vi "svx_Waterfall Execute.vi"(0 "Data In":T2={"z0"=0.0, "dz"=1.0, "Plots"=[]}, 1 "Display State In":T6={"X Scale Width %"=50.0, "Y Scale Height %"=50.0, "X-Axis Range"={"Minimum"=0.0, "Maximum"=10.0}, "Y-Axis Range"={"Minimum"=0.0, "Maximum"=10.0}, "Z-Axis Range"={"Minimum"=0.0, "Maximum"=10.0}, "Plot Color"=61212, "Frame Color"=16252785, "Background Color"=16777222, "Initial AutoScale Y"=TRUE, "AutoScale X"=2, "AutoScale Y"=2, "AutoScale Z"=2, "Plot Transparency"=FALSE, "X-Axis Name"="Frequency", "Y-Axis Name"="Amplitude", "Z-Axis Name"="", "X-Axis Scaling Factor"={"Offset"=0.0, "Multiplier"=1.0}, "Y-Axis Scaling Factor"={"Offset"=0.0, "Multiplier"=1.0}, "Z-Axis Scaling Factor"={"Offset"=0.0, "Multiplier"=1.0}, "X-Scale Visible"=TRUE, "Y-Scale Visible"=TRUE, "Z-Scale Visible"=TRUE, "X-Scale Label Visible"=TRUE, "Y-Scale Label Visible"=TRUE, "Z-Scale Label Visible"=TRUE, "X-Axis Range Scaled"={"Minimum"=0.0, "Maximum"=10.0}, "Y-Axis Range Scaled"={"Minimum"=0.0, "Maximum"=10.0}, "Z-Axis Range Scaled"={"Minimum"=0.0, "Maximum"=10.0}, "Rev Z Order"=FALSE, "X-Scale Format Str"="%#.4g", "Y-Scale Format Str"="%#.4g", "Z-Scale Format Str"="%#.4g", "Decor color"=12369084, "Scale Range Change"=refnum, "out of state queue"=refnum, "property nodes"=refnum, "Lines"=[], "Line Properties"={"Line Color"=61212, "Line Width"=61212, "Line Style"=enum."Dash", "DisplayLines"=FALSE}} {"Line Properties"."Line Width" min=1}, 2 "Container State":T7, 4 "Dec/Cropped and Lines":T1={"Dec/Cropped in"={"z0"=0.0, "dz"=1.0, "Plots"=[]}, "Lines"=[]}, 6 "Execution Tasks":T5[](array[typedef]), 7 "XY Graph Ref":refnum<vi>, 8 "Coords":T4, 9 "XY Scale Graph ref":refnum<vi>, 11 "Z Scale Graph ref":refnum<vi>, 12 "This VI":refnum<vi>, 13 "Background ref":refnum<vi>) -> (14 "Data Out":T2={"z0"=0.0, "dz"=1.0, "Plots"=[]}, 15 "Display State Out":T6={"X Scale Width %"=50.0, "Y Scale Height %"=50.0, "X-Axis Range"={"Minimum"=0.0, "Maximum"=10.0}, "Y-Axis Range"={"Minimum"=0.0, "Maximum"=10.0}, "Z-Axis Range"={"Minimum"=0.0, "Maximum"=10.0}, "Plot Color"=61212, "Frame Color"=16252785, "Background Color"=16777222, "Initial AutoScale Y"=TRUE, "AutoScale X"=2, "AutoScale Y"=2, "AutoScale Z"=2, "Plot Transparency"=FALSE, "X-Axis Name"="Frequency", "Y-Axis Name"="Amplitude", "Z-Axis Name"="", "X-Axis Scaling Factor"={"Offset"=0.0, "Multiplier"=1.0}, "Y-Axis Scaling Factor"={"Offset"=0.0, "Multiplier"=1.0}, "Z-Axis Scaling Factor"={"Offset"=0.0, "Multiplier"=1.0}, "X-Scale Visible"=TRUE, "Y-Scale Visible"=TRUE, "Z-Scale Visible"=TRUE, "X-Scale Label Visible"=TRUE, "Y-Scale Label Visible"=TRUE, "Z-Scale Label Visible"=TRUE, "X-Axis Range Scaled"={"Minimum"=0.0, "Maximum"=10.0}, "Y-Axis Range Scaled"={"Minimum"=0.0, "Maximum"=10.0}, "Z-Axis Range Scaled"={"Minimum"=0.0, "Maximum"=10.0}, "Rev Z Order"=FALSE, "X-Scale Format Str"="%#.4g", "Y-Scale Format Str"="%#.4g", "Z-Scale Format Str"="%#.4g", "Decor color"=12369084, "Scale Range Change"=refnum, "out of state queue"=refnum, "property nodes"=refnum, "Lines"=[], "Line Properties"={"Line Color"=61212, "Line Width"=61212, "Line Style"=enum."Dash", "DisplayLines"=FALSE}} {"Line Properties"."Line Width" min=1}, 18 "Dec/Cropped out":T1={"Dec/Cropped in"={"z0"=0.0, "dz"=1.0, "Plots"=[]}, "Lines"=[]})   [LabVIEW 2017, in "SVX Waterfall Graph.xctl"]
uses:
  <vilib>/addons/_XControls/Waterfall Graph/SVX Waterfall Graph.xctl
  <vilib>/addons/_XControls/Waterfall Graph/subVIs/svx_Waterfall State.ctl
  <vilib>/addons/_NISVFA/_Shared subVIs/Controls/svc_Cluster of Array of Cluster of XYZ.ctl
  <vilib>/_xctls/Container State.ctl
  <vilib>/addons/_XControls/Waterfall Graph/subVIs/svx_Waterfall Data.ctl
  <vilib>/addons/_XControls/Waterfall Graph/subVIs/svx_Waterfall Execution Tasks.ctl
  <vilib>/Utility/miscctls.llb/LVPoint32TypeDef.ctl
  <vilib>/addons/_XControls/Waterfall Graph/subVIs/svx_CroppedData.ctl
  <vilib>/_xctls/XControlSupport.lvlib
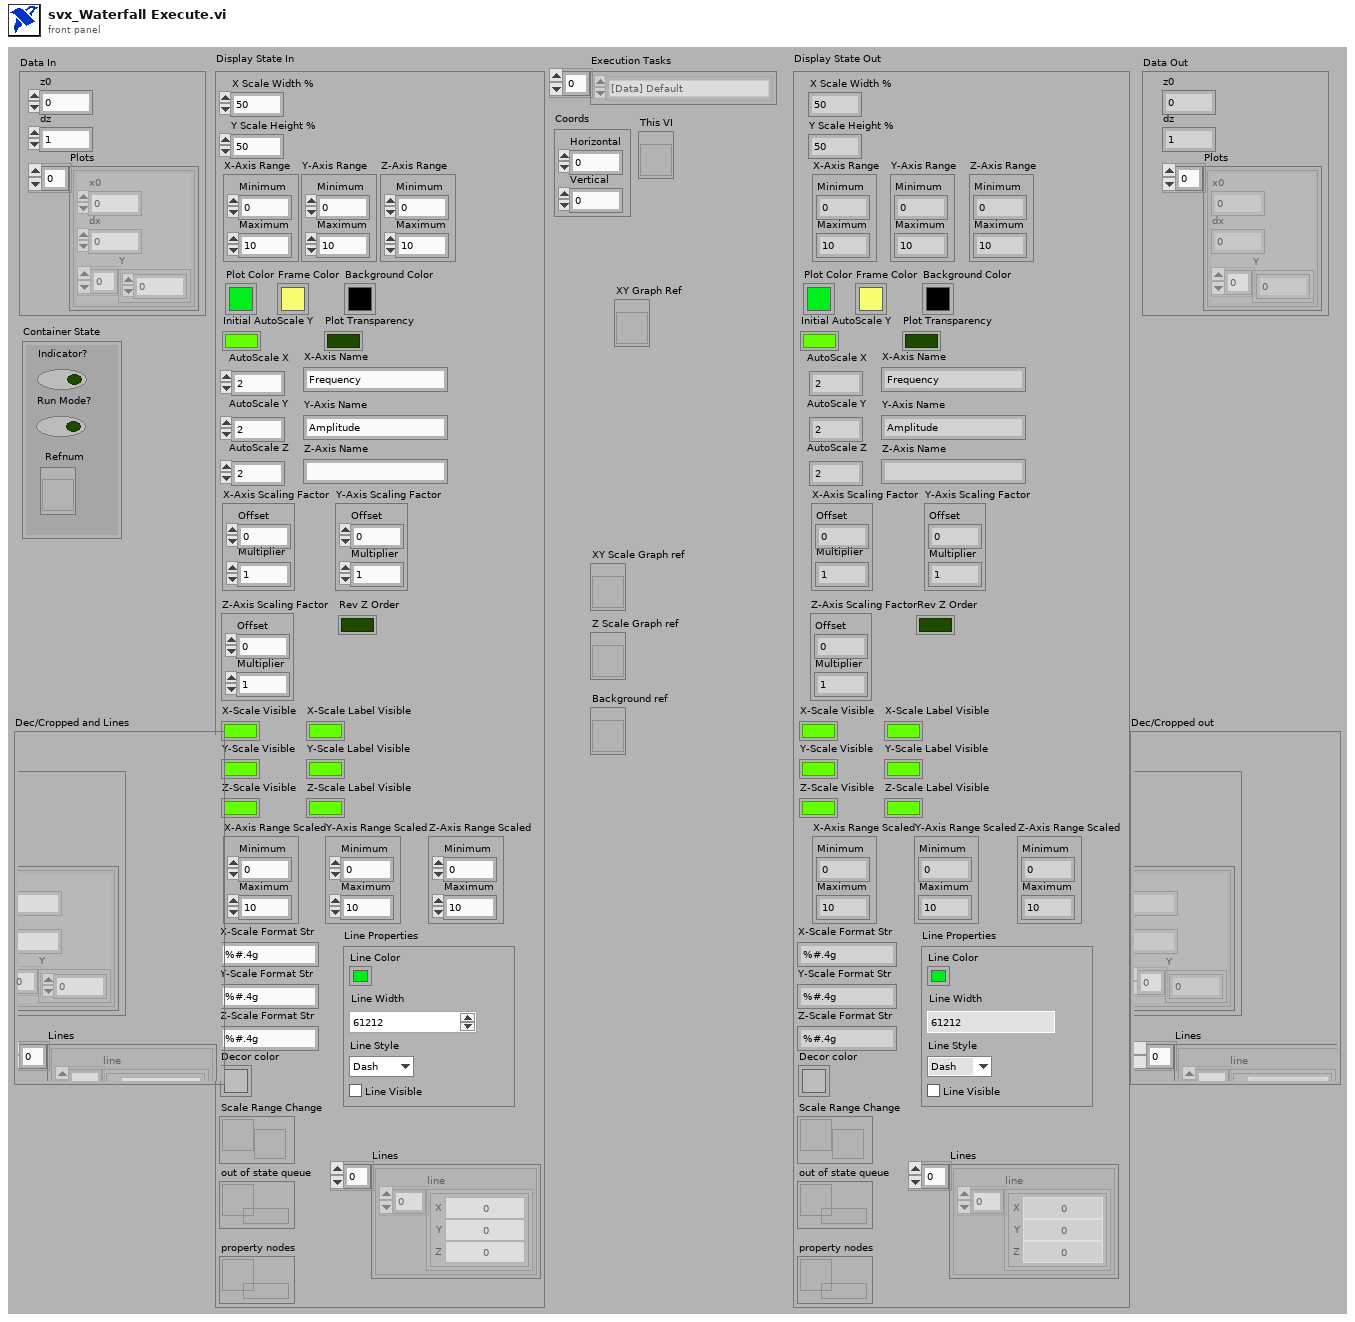
[diagram p1: front panel]
types:
  T1 = typedef "SVX Waterfall Graph.xctl/svx_CroppedData.ctl" = cluster{"Dec/Cropped in":T2, "Lines":T3[]}
  T2 = typedef "SVX Waterfall Graph.xctl/svx_Waterfall Data.ctl" = cluster{"z0":dbl, "dz":dbl, "Plots":cluster{"x0":dbl, "dx":dbl, "Y":dbl[]}[]}
  T3 = typedef "svc_Cluster of Array of Cluster of XYZ.ctl" = cluster{"line":cluster{"X":dbl, "Y":dbl, "Z":dbl}[]}
  T4 = typedef "LVPoint32TypeDef.ctl" = cluster{"Horizontal":i32, "Vertical":i32}
  T5 = typedef "SVX Waterfall Graph.xctl/svx_Waterfall Execution Tasks.ctl" = enum16{"[Data] Default", "[Data] Update Graph", "[Pane] Calculate Size from Coord Change", "[Pane] Calculate Size from Display State", "[Plot] Redraw Frame", "[Plot] Update Plot Color", "[Scale] Autoscale or Crop X, Y, Z", "[Scale] Resize Scales", "[Scale] Align Scale Labels", "[Plot] Initialize Plot", "[Scale] X Scale", "[Scale] Y Scale", "[Scale] Z Scale", "[Scale] Multiplier/Offset", "[Scale] Name", "[Scale] Visible", "[Scale] Label Visible", "[Scale] Format"}
  T6 = typedef "SVX Waterfall Graph.xctl/svx_Waterfall State.ctl" = cluster{"X Scale Width %":dbl, "Y Scale Height %":dbl, "X-Axis Range":cluster{"Minimum":dbl, "Maximum":dbl}, "Y-Axis Range":cluster{"Minimum":dbl, "Maximum":dbl}, "Z-Axis Range":cluster{"Minimum":dbl, "Maximum":dbl}, "Plot Color":u32, "Frame Color":u32, "Background Color":u32, "Initial AutoScale Y":bool, "AutoScale X":u8, "AutoScale Y":u8, "AutoScale Z":u8, "Plot Transparency":bool, "X-Axis Name":string, "Y-Axis Name":string, "Z-Axis Name":string, "X-Axis Scaling Factor":cluster{"Offset":dbl, "Multiplier":dbl}, "Y-Axis Scaling Factor":cluster{"Offset":dbl, "Multiplier":dbl}, "Z-Axis Scaling Factor":cluster{"Offset":dbl, "Multiplier":dbl}, "X-Scale Visible":bool, "Y-Scale Visible":bool, "Z-Scale Visible":bool, "X-Scale Label Visible":bool, "Y-Scale Label Visible":bool, "Z-Scale Label Visible":bool, "X-Axis Range Scaled":cluster{"Minimum":dbl, "Maximum":dbl}, "Y-Axis Range Scaled":cluster{"Minimum":dbl, "Maximum":dbl}, "Z-Axis Range Scaled":cluster{"Minimum":dbl, "Maximum":dbl}, "Rev Z Order":bool, "X-Scale Format Str":string, "Y-Scale Format Str":string, "Z-Scale Format Str":string, "Decor color":u32, "Scale Range Change":refnum<user-event>, "out of state queue":refnum<queue>, "property nodes":refnum<queue>, "Lines":T3[], "Line Properties":cluster{"Line Color":u32, "Line Width":u16, "Line Style":enum32{"Solid", "Dash", "Dot", "DashDot", "DashDotDot"}, "DisplayLines":bool}}
  T7 = typedef "XControlSupport.lvlib/Container State.ctl" = cluster{"Indicator?":bool, "Run Mode?":bool, " Refnum":refnum<vi>}
  T8 = enum16{"coerce to nearest", "coerce to next highest", "coerce to next lowest", "interpolate"}
  T9 = cluster{"Amp Width":u32, "Amp Height":u32, "Z Height":u32, "Wform Height":u32, "Wform Width":u32}
  T10 = cluster{"Width":u16, "Style":enum32{"Solid", "Dash", "Dot", "DashDot", "DashDotDot"}}
  T11 = typedef "LVRectTypeDef.ctl" = cluster{"Left":i16, "Top":i16, "Right":i16, "Bottom":i16}
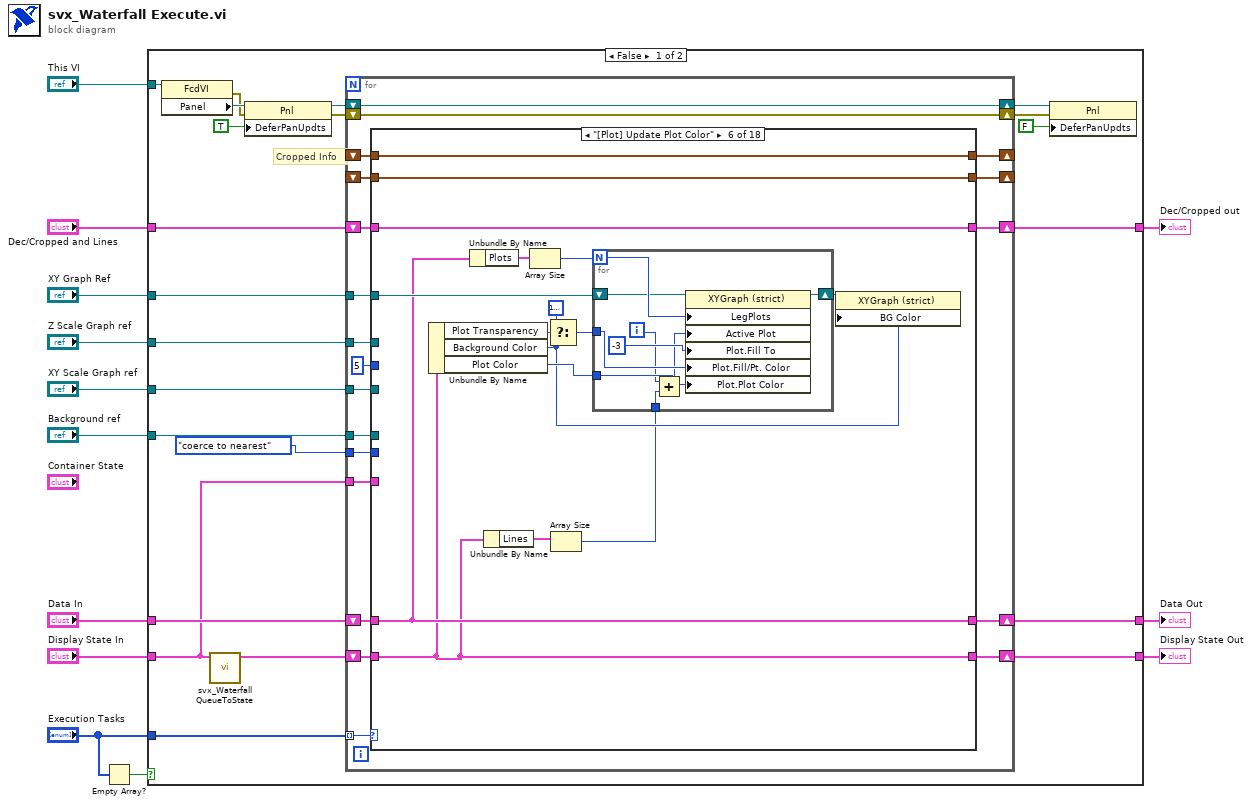
[diagram p0: block diagram]
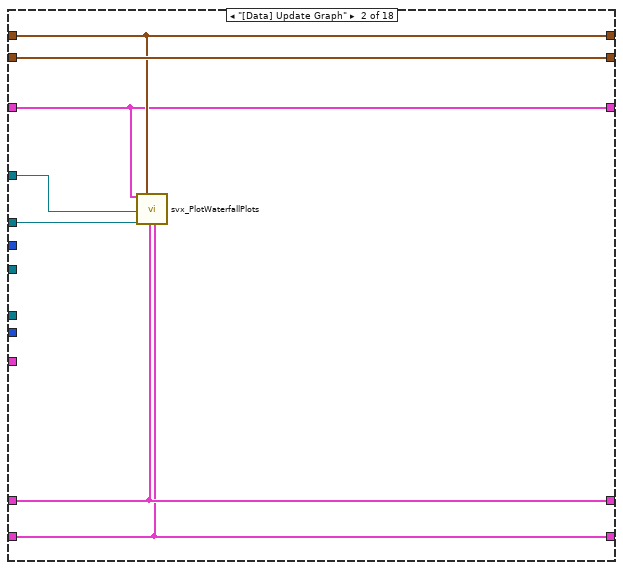
[diagram p3: hidden frame]
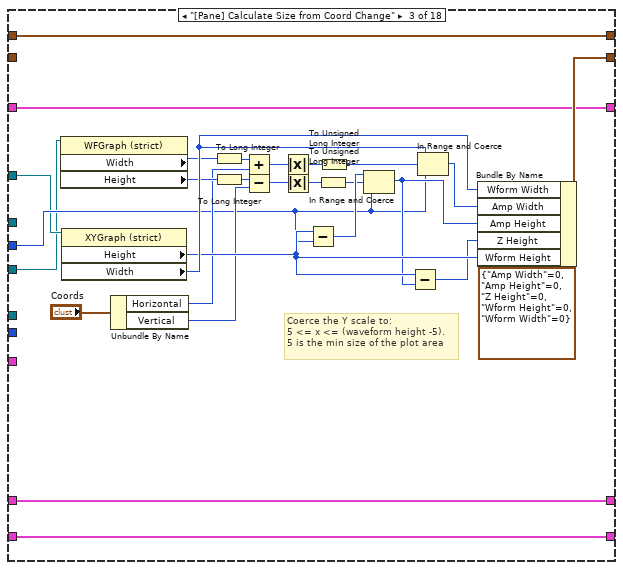
[diagram p4: hidden frame]
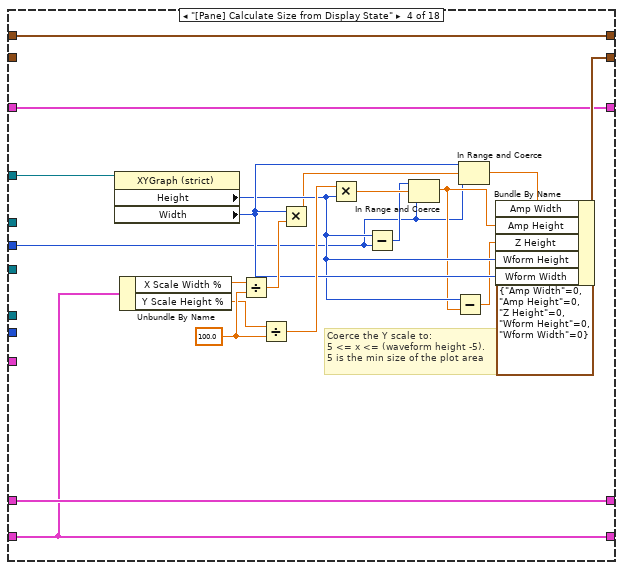
[diagram p5: hidden frame]
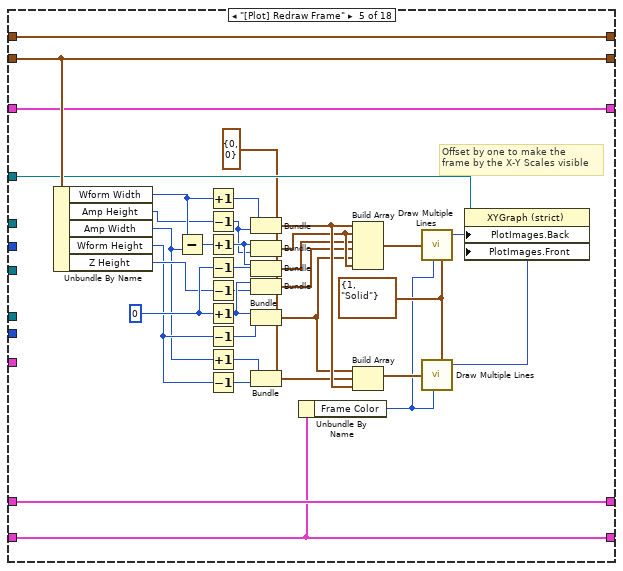
[diagram p6: hidden frame]
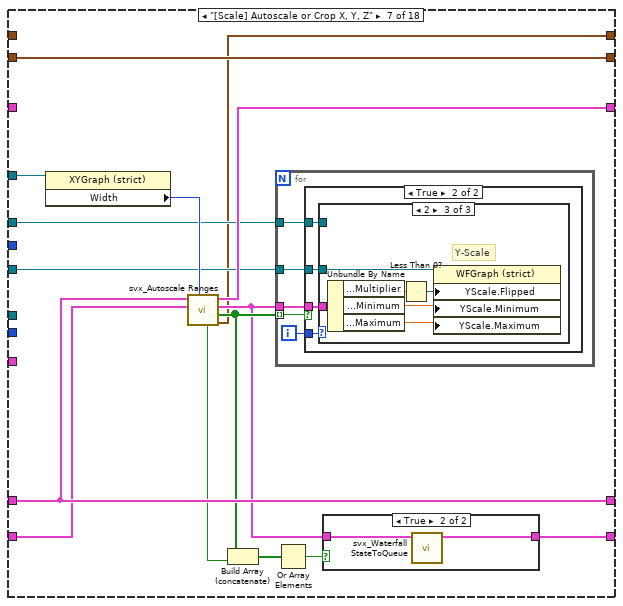
[diagram p7: hidden frame]
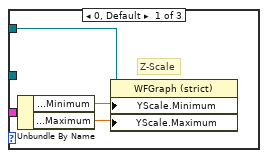
[diagram p9: hidden frame]
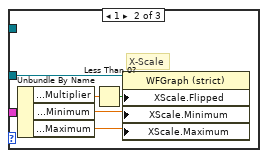
[diagram p10: hidden frame]
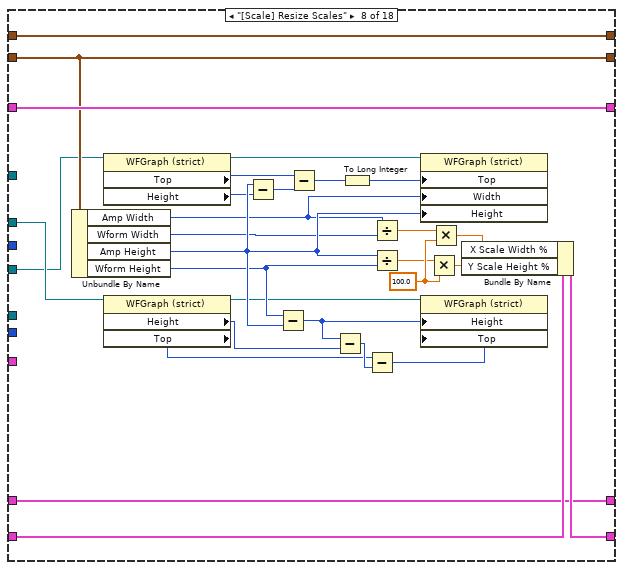
[diagram p12: hidden frame]
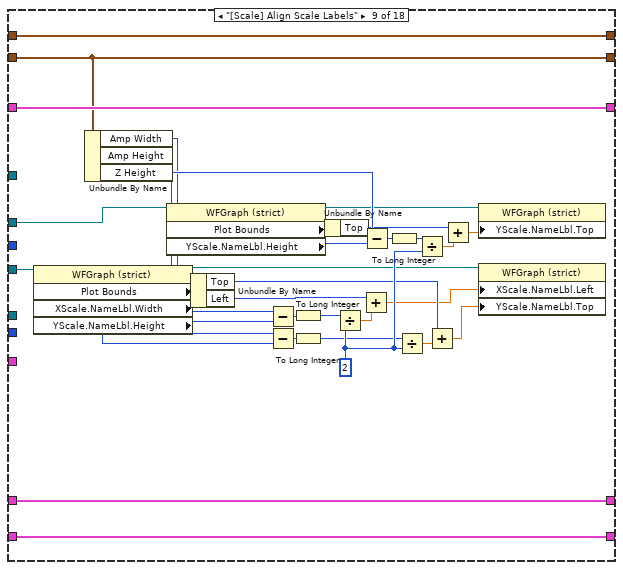
[diagram p13: hidden frame]
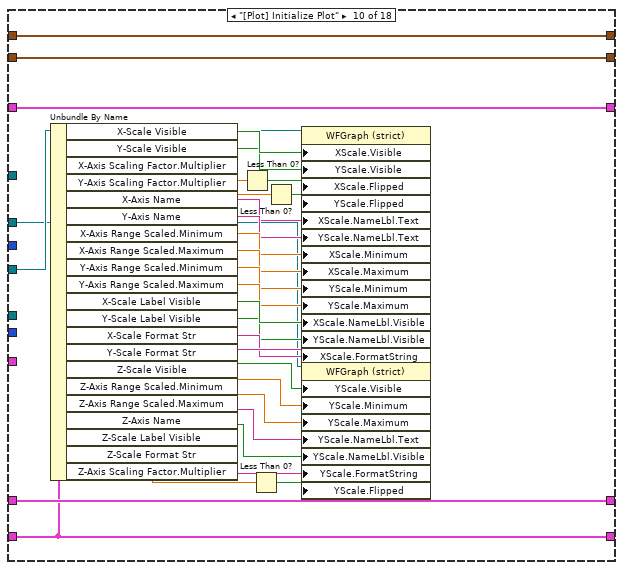
[diagram p14: hidden frame]
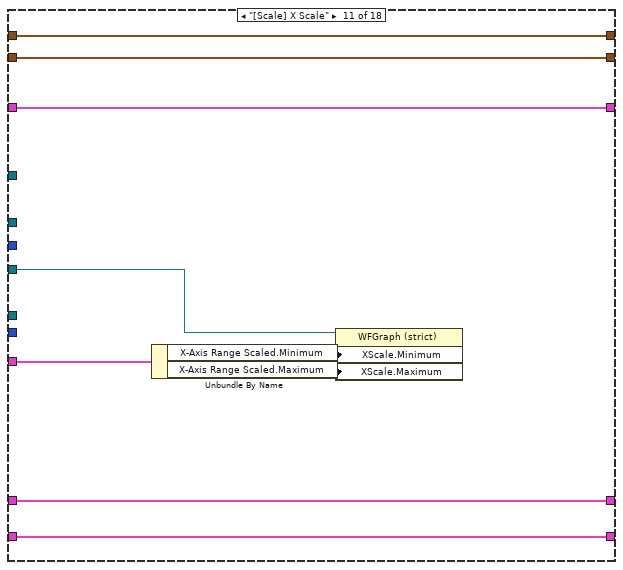
[diagram p15: hidden frame]
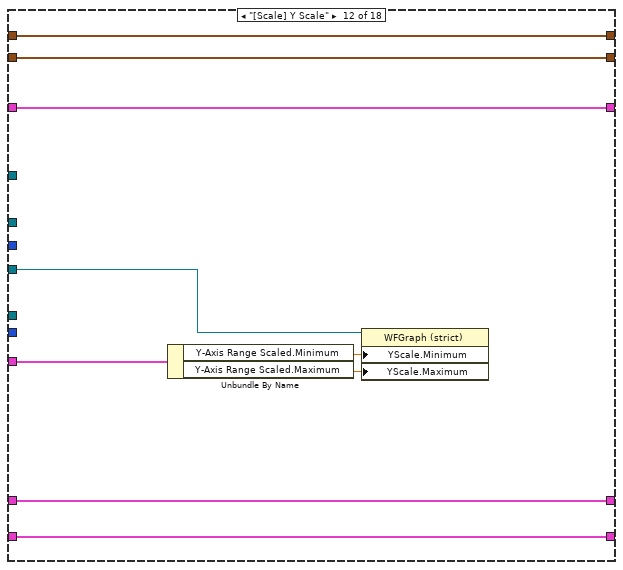
[diagram p16: hidden frame]
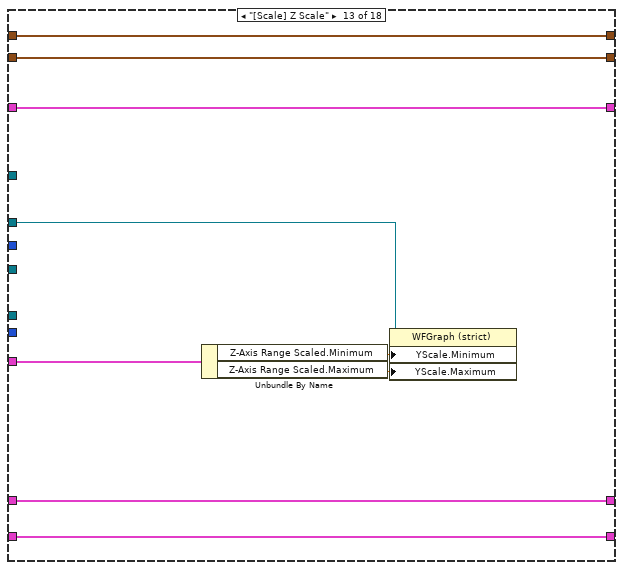
[diagram p17: hidden frame]
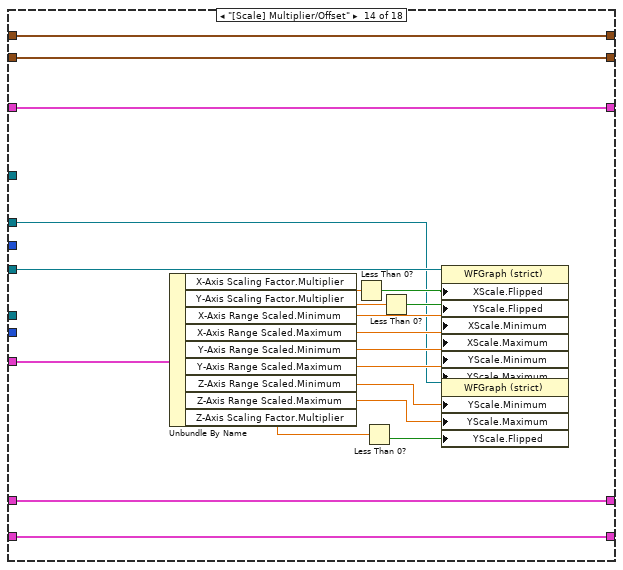
[diagram p18: hidden frame]
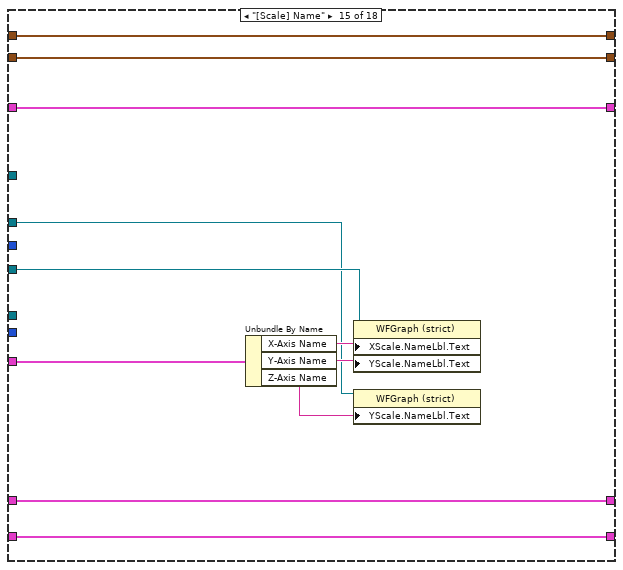
[diagram p19: hidden frame]
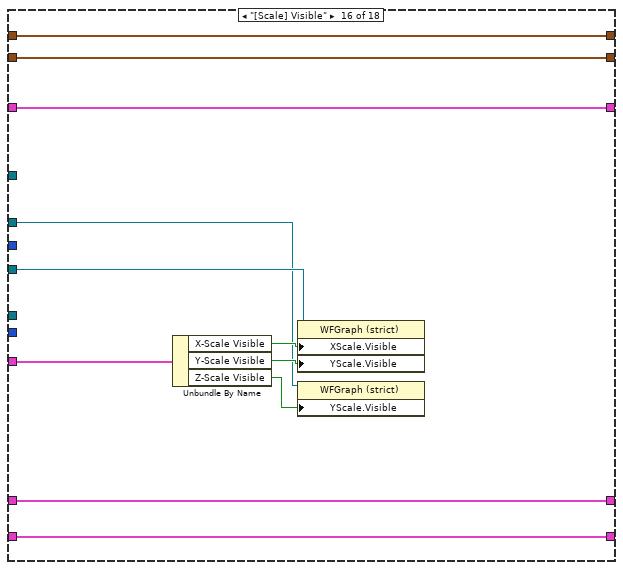
[diagram p20: hidden frame]
diagram:
  n1 = Empty Array?(array="Execution Tasks") -> (empty?=w3:bool)
  n2 = case shown="False" w3 {
    tunnel: "This VI" -> [w32 _]
    tunnel: "XY Graph Ref" -> [w26 _]
    tunnel: "Z Scale Graph ref" -> [w25 _]
    tunnel: "XY Scale Graph ref" -> [w24 _]
    tunnel: "Execution Tasks" -> [w23 _]
    tunnel: "Data In" -> [w22 w405]
    tunnel: [w21 w405] -> w9
    tunnel: [w19 w406] -> w8
    tunnel: "Dec/Cropped and Lines" -> [w18 w404]
    tunnel: [w17 w404] -> w6
    tunnel: "Background ref" -> [w16 _]
    tunnel: "Display State In" -> [w15 w406]
    frame False {
      # "Cropped Info"
      n3 = property class="FcdVI"(reference=w32) -> (error out=w33:errorcluster, "Panel"=w35:refnum<vi>)  [unwired: 1 in, 1 out]
      n4 = call <vilib>:"svx_Waterfall QueueToState.vi"("State In"=w15) -> ("State Out"=w20:T6)  [unwired: 10 in]
      n5 = property class="Pnl"(reference=w35, error in=w33, "DeferPanUpdts"=TRUE ("Defer Panel Updates")) -> (reference out=w31:refnum<vi>, error out=w30:errorcluster)
      n6 = for {
        shift-right: [w55] -> w27
        shift-left: w31 -> [w55]
        shift-right: [w54] -> w28
        shift-left: w30 -> [w54]
        tunnel: w26 -> [w48]
        tunnel: w25 -> [w46]
        tunnel: w24 -> [w45]
        tunnel: w23 -> [w53] mode=indexing
        shift-right: [w51] -> w21
        shift-left: w22 -> [w52]
        shift-right: [w49] -> w19
        shift-left: w20 -> [w50]
        shift-right: [w44] -> _
        shift-left: _ -> [w43]
        shift-right: [w41] -> w17
        shift-left: w18 -> [w42]
        shift-right: [w40] -> _
        shift-left: _ -> [w39]
        tunnel: w16 -> [w38]
        tunnel: w15 -> [w37]
        tunnel: T8."coerce to nearest" ("frequency coercion") -> [w36]
        n7 = case shown="\"[Plot] Update Plot Color\"" w53 {
          tunnel: w52 -> [w60 w66 w79 w116 w123 w159 w188 w225 w281 w287 w318 w327 w336 w356 w367 w378 w389 w400]
          tunnel: [w60 w66 w79 w116 w123 w159 w188 w225 w281 w287 w318 w327 w336 w356 w367 w378 w389 w400] -> w51
          tunnel: w50 -> [w59 w65 w78 w99 w122 w155 w187 w227 w280 w286 w313 w323 w332 w355 w366 w377 w385 w399]
          tunnel: [w59 w65 w78 w99 w122 w155 w183 w226 w280 w286 w313 w323 w332 w355 w366 w377 w385 w399] -> w49
          tunnel: w48 -> [_ w62 w77 w101 w118 w160 w190 _ _ _ _ _ _ _ _ _ _ _]
          tunnel: u32 5 ("Plot Area:Size:Height") -> [_ _ w80 w100 _ _ _ _ _ _ _ _ _ _ _ _ _ _]
          tunnel: w46 -> [_ w63 _ _ _ _ w179 w223 w252 w285 _ _ w333 w340 w360 w371 w383 w393]
          tunnel: w45 -> [_ _ w72 _ _ _ w178 w220 w249 w288 w315 w324 _ w341 w361 w372 w384 w394]
          tunnel: [w58 w67 w75 w98 w121 w157 w191 w222 w251 w283 w320 w329 w338 w358 w369 w380 w391 w402] -> w44
          tunnel: w43 -> [w58 w67 _ _ w121 w157 w191 w222 w251 w283 w320 w329 w338 w358 w369 w380 w391 w402]
          tunnel: w42 -> [w57 w61 w74 w97 w120 w158 _ w224 w279 w282 w319 w328 w337 w357 w368 w379 w390 w401]
          tunnel: [w57 w61 w74 w97 w120 w158 w180 w224 w279 w282 w319 w328 w337 w357 w368 w379 w390 w401] -> w41
          tunnel: [w56 w64 w73 w96 w119 w156 w177 w221 w278 w284 w321 w330 w339 w359 w370 w381 w392 w403] -> w40
          tunnel: w39 -> [w56 w64 w73 w96 w119 w156 _ w221 w278 w284 w321 w330 w339 w359 w370 w381 w392 w403]
          tunnel: w38 -> [_ _ _ _ _ _ _ _ _ _ _ _ _ _ _ _ _ _]
          tunnel: w37 -> [_ _ _ _ _ _ _ _ _ _ w314 w322 w331 w342 w362 w373 w382 w395]
          tunnel: w36 -> [_ _ _ _ _ _ _ _ _ _ _ _ _ _ _ _ _ _]
          frame "[Data] Default", Default {
          }
          frame "[Data] Update Graph" {
            n8 = call <vilib>:"svx_PlotWaterfallPlots.vi"("Dec/Cropped in"=w61, "XYGraph in"=w62, "Z Scale Graph ref"=w63, "Cropped Info in"=w64, "Data In"=w66, "State Out"=w65) -> ()  [unwired: 14 in]
          }
          frame "[Pane] Calculate Size from Coord Change" {
            # "Coerce the Y scale to:\n5 <= x <= (waveform height -5).\n5 is the min size of the plot area"
            n9 = property on="Property Node" class="WFGraph (strict)"(reference=w72) -> ("Width"=w88:u32, "Height"=w84:u32)  [unwired: 1 in, 2 out]
            n10 = property on="Property Node" class="XYGraph (strict)"(reference=w77) -> ("Height"=w94:u32, "Width"=w95:u32)  [unwired: 1 in, 2 out]
            n11 = Unbundle By Name("Coords") -> ("Horizontal"=w81:i32, "Vertical"=w85:i32)
            n12 = To Long Integer(number=w88) -> (32bit integer=w87:i32)
            n13 = To Long Integer(number=w84) -> (32bit integer=w86:i32)
            n14 = Add(x=w87, y=w81) -> (x+y=w89:i32)
            n15 = Subtract(x=w86, y=w85) -> (x-y=w82:i32)
            n16 = Absolute Value(x=w89) -> (abs(x)=w71:i32)
            n17 = Absolute Value(x=w82) -> (abs(x)=w69:i32)
            n18 = Subtract(x=w94, y=w80) -> (x-y=w83:u32)
            n19 = To Unsigned Long Integer(number=w69) -> (unsigned 32bit integer=w68:u32)
            n20 = To Unsigned Long Integer(number=w71) -> (unsigned 32bit integer=w70:u32)
            n21 = In Range and Coerce(upper limit=w83, x=w68, lower limit=w80) -> (coerced(x)=w91:u32)  [unwired: 1 out]
            n22 = Subtract(x=w94, y=w91) -> (x-y=w92:u32)
            n23 = In Range and Coerce(upper limit=w95, x=w70, lower limit=w80) -> (coerced(x)=w90:u32)  [unwired: 1 out]
            n24 = Bundle By Name(cluster=T9 {"Amp Width"=0, "Amp Height"=0, "Z Height"=0, "Wform Height"=0, "Wform Width"=0}, "Wform Width"=w95, "Amp Width"=w90, "Amp Height"=w91, "Z Height"=w92, "Wform Height"=w94) -> (w75:T9)
          }
          frame "[Pane] Calculate Size from Display State" {
            w115 = 100.0 ("y")
            # "Coerce the Y scale to:\n5 <= x <= (waveform height -5).\n5 is the min size of the plot area"
            n25 = property on="Property Node" class="XYGraph (strict)"(reference=w101) -> ("Height"=w109:u32, "Width"=w110:u32)  [unwired: 1 in, 2 out]
            n26 = Unbundle By Name(w99) -> ("X Scale Width %"=w113:dbl, "Y Scale Height %"=w111:dbl)
            n27 = Divide(x=w113, y=w115) -> (x/y=w114:dbl)
            n28 = Divide(x=w111, y=w115) -> (x/y=w112:dbl)
            n29 = Multiply(x=w110, y=w114) -> (x*y=w105:dbl)
            n30 = Multiply(x=w112, y=w109) -> (x*y=w104:dbl)
            n31 = Subtract(x=w109, y=w100) -> (x-y=w102:u32)
            n32 = In Range and Coerce(upper limit=w102, x=w104, lower limit=w100) -> (coerced(x)=w107:dbl)  [unwired: 1 out]
            n33 = Subtract(x=w109, y=w107) -> (x-y=w108:dbl)
            n34 = In Range and Coerce(upper limit=w110, x=w105, lower limit=w100) -> (coerced(x)=w106:dbl)  [unwired: 1 out]
            n35 = Bundle By Name(cluster=T9 {"Amp Width"=0, "Amp Height"=0, "Z Height"=0, "Wform Height"=0, "Wform Width"=0}, "Amp Width"=w106, "Amp Height"=w107, "Z Height"=w108, "Wform Height"=w109, "Wform Width"=w110) -> (w98:T9)
          }
          frame "[Plot] Redraw Frame" {
            w117 = cluster{"x":i16, "y":i16} {"x"=0, "y"=0} ("cluster")
            w151 = T10 {"Width"=1, "Style"=enum."Solid"} ("pen")
            w145 = u32 0 ("Offset")
            # "Offset by one to make the\nframe by the X-Y Scales visible"
            n36 = Unbundle By Name(w121) -> ("Wform Width"=w138:u32, "Amp Height"=w136:u32, "Amp Width"=w132:u32, "Wform Height"=w134:u32, "Z Height"=w143:u32)
            n37 = Subtract(x=w138, y=w132) -> (x-y=w140:u32)
            n38 = Increment(x=w138) -> (x+1=w139:u32)
            n39 = Decrement(x=w136) -> (x-1=w137:u32)
            n40 = Increment(x=w140) -> (x+1=w141:u32)
            n41 = Decrement(x=w145) -> (x-1=w144:u32)
            n42 = Decrement(x=w143) -> (x-1=w142:u32)
            n43 = Increment(x=w145) -> (x+1=w146:u32)
            n44 = Decrement(x=w134) -> (x-1=w131:u32)
            n45 = Increment(x=w132) -> (x+1=w133:u32)
            n46 = Decrement(x=w134) -> (x-1=w135:u32)
            n47 = Bundle(cluster=w117, "x"=w139, "y"=w137) -> (w130:cluster{"x":i16, "y":i16})
            n48 = Bundle(cluster=w117, "x"=w141, "y"=w137) -> (w129:cluster{"x":i16, "y":i16})
            n49 = Bundle(cluster=w117, "x"=w141, "y"=w144) -> (w125:cluster{"x":i16, "y":i16})
            n50 = Bundle(cluster=w117, "x"=w146, "y"=w142) -> (w126:cluster{"x":i16, "y":i16})
            n51 = Bundle(cluster=w117, "x"=w146, "y"=w131) -> (w128:cluster{"x":i16, "y":i16})
            n52 = Bundle(cluster=w117, "x"=w133, "y"=w135) -> (w127:cluster{"x":i16, "y":i16})
            n53 = Unbundle By Name(w122) -> ("Frame Color"=w124:u32)
            n54 = Build Array(w130, w129, w125, w126, w128, w129) -> (w147:cluster{"x":i16, "y":i16}[])
            n55 = Build Array(w128, w127, w130) -> (w148:cluster{"x":i16, "y":i16}[])
            n56 = call <vilib>:"Draw Multiple Lines.vi"("line endpoints"=w147, "color(black)"=w124, "pen"=w151) -> ("new picture"=w149:picture)  [unwired: 6 in]
            n57 = call <vilib>:"Draw Multiple Lines.vi"("line endpoints"=w148, "color(black)"=w124, "pen"=w151) -> ("new picture"=w150:picture)  [unwired: 6 in]
            n58 = property on="Property Node" class="XYGraph (strict)"(reference=w118, "PlotImages.Back"=w149, "PlotImages.Front"=w150) -> ()  [unwired: 1 in, 2 out]
          }
          frame "[Plot] Update Plot Color" {
            n59 = Unbundle By Name(w155) -> ("Plot Transparency"=w163:bool, "Background Color"=w162:u32, "Plot Color"=w166:u32)
            n60 = Unbundle By Name(w159) -> ("Plots"=w161:cluster{"x0":dbl, "dx":dbl, "Y":dbl[]}[])
            n61 = Unbundle By Name(w155) -> ("Lines"=w154:T3[])
            n62 = Array Size(array=w161) -> (size(s)=w152:i32)
            n63 = Select(t=u32 16777216, s=w163, f=w162) -> (s? t:f=w164:u32)
            n64 = Array Size(array=w154) -> (size(s)=w153:i32)
            n65 = for {
              N: w152 -> [w173]
              tunnel: w164 -> [w175]
              tunnel: w166 -> [w174]
              shift-right: [w171] -> w167
              shift-left: w160 -> [w172]
              tunnel: w153 -> [w170]
              i -> [w169]
              n66 = Add(x=w169, y=w170) -> (x+y=w168:i32)
              n67 = property on="Property Node" class="XYGraph (strict)"(reference=w172, "LegPlots"=w173, "Active Plot"=w168, "Plot.Fill To"=i16 -3, "Plot.Fill/Pt. Color"=w175, "Plot.Plot Color"=w174) -> (reference out=w171:refnum<vi>)  [unwired: 1 in, 1 out]
            }
            n68 = property on="Property Node" class="XYGraph (strict)"(reference=w167, "BG Color"=w162) -> ()  [unwired: 1 in, 2 out]
          }
          frame "[Scale] Autoscale or Crop X, Y, Z" {
            n69 = property on="Property Node" class="XYGraph (strict)"(reference=w190) -> ("Width"=w189:u32)  [unwired: 1 in, 2 out]
            n70 = call <vilib>:"svx_Autoscale Ranges.vi"("Plot Area:Size:Width"=w189, "Display State In"=w187, "Data Array In"=w188) -> ("Cropped Info out"=w177:cluster{"First Index":i32, "Length":i32}, "Update Ranges"=w182:bool[], "Display State Out"=w181:T6, "Dec/Cropped and Lines Out"=w180:T1, "Update Autoscale"=w184:bool)  [unwired: 4 in]
            n71 = Build Array (concatenate)(w182, w184) -> (w185:bool[])
            n72 = for {
              tunnel: w182 -> [w196] mode=indexing
              tunnel: w181 -> [w194]
              tunnel: w179 -> [w193]
              tunnel: w178 -> [w192]
              i -> [w195]
              n73 = case shown="True" w196 {
                tunnel: w195 -> [_ w200]
                tunnel: w194 -> [_ w199]
                tunnel: w193 -> [_ w198]
                tunnel: w192 -> [_ w197]
                frame False {
                }
                frame True {
                  n74 = case shown="2" w200 {
                    tunnel: w199 -> [w204 w210 w216]
                    tunnel: w198 -> [w201 _ _]
                    tunnel: w197 -> [_ w205 w211]
                    frame 0, Default {
                      # "Z-Scale"
                      n75 = Unbundle By Name(w204) -> ("Z-Axis Range Scaled.Minimum"=w203:dbl, "Z-Axis Range Scaled.Maximum"=w202:dbl)
                      n76 = property on="Property Node" class="WFGraph (strict)"(reference=w201, "YScale.Minimum"=w203, "YScale.Maximum"=w202) -> ()  [unwired: 1 in, 2 out]
                    }
                    frame 1 {
                      # "X-Scale"
                      n77 = Unbundle By Name(w210) -> ("X-Axis Scaling Factor.Multiplier"=w209:dbl, "X-Axis Range Scaled.Minimum"=w207:dbl, "X-Axis Range Scaled.Maximum"=w206:dbl)
                      n78 = Less Than 0?(x=w209) -> (x < 0?=w208:bool)
                      n79 = property on="Property Node" class="WFGraph (strict)"(reference=w205, "XScale.Flipped"=w208, "XScale.Minimum"=w207, "XScale.Maximum"=w206) -> ()  [unwired: 1 in, 2 out]
                    }
                    frame 2 {
                      # "Y-Scale"
                      n80 = Unbundle By Name(w216) -> ("Y-Axis Scaling Factor.Multiplier"=w215:dbl, "Y-Axis Range Scaled.Minimum"=w213:dbl, "Y-Axis Range Scaled.Maximum"=w212:dbl)
                      n81 = Less Than 0?(x=w215) -> (x < 0?=w214:bool)
                      n82 = property on="Property Node" class="WFGraph (strict)"(reference=w211, "YScale.Flipped"=w214, "YScale.Minimum"=w213, "YScale.Maximum"=w212) -> ()  [unwired: 1 in, 2 out]
                    }
                  }
                }
              }
            }
            n83 = Or Array Elements(Boolean array=w185) -> (logical OR=w186:bool)
            n84 = case shown="True" w186 {
              tunnel: w181 -> [w217 w219]
              tunnel: [w217 w218] -> w183
              frame False {
              }
              frame True {
                n85 = call <vilib>:"svx_Waterfall StateToQueue.vi"("Display State In"=w219) -> ("Display State Out"=w218:T6)  [unwired: 10 in]
              }
            }
          }
          frame "[Scale] Resize Scales" {
            w242 = 100.0 ("x/y")
            n86 = Unbundle By Name(w222) -> ("Amp Width"=w243:u32, "Wform Width"=w239:u32, "Amp Height"=w244:u32, "Wform Height"=w238:u32)
            n87 = property on="Property Node" class="WFGraph (strict)"(reference=w220) -> (reference out=w229:refnum<vi>, "Top"=w234:i32, "Height"=w237:u32)  [unwired: 1 in, 1 out]
            n88 = property on="Property Node" class="WFGraph (strict)"(reference=w223) -> (reference out=w228:refnum<vi>, "Height"=w230:u32, "Top"=w231:i32)  [unwired: 1 in, 1 out]
            n89 = Subtract(x=w244, y=w237) -> (x-y=w235:u32)
            n90 = Subtract(x=w238, y=w244) -> (x-y=w236:u32)
            n91 = Subtract(x=w234, y=w235) -> (x-y=w245:u32)
            n92 = Subtract(x=w236, y=w230) -> (x-y=w232:u32)
            n93 = To Long Integer(number=w245) -> (32bit integer=w246:i32)
            n94 = Subtract(x=w231, y=w232) -> (x-y=w233:u32)
            n95 = Divide(x=w243, y=w239) -> (x/y=w241:dbl)
            n96 = Divide(x=w244, y=w238) -> (x/y=w240:dbl)
            n97 = property on="Property Node" class="WFGraph (strict)"(reference=w229, "Top"=w246, "Width"=w243, "Height"=w244) -> ()  [unwired: 1 in, 2 out]
            n98 = property on="Property Node" class="WFGraph (strict)"(reference=w228, "Height"=w236, "Top"=w233) -> ()  [unwired: 1 in, 2 out]
            n99 = Multiply(x=w240, y=w242) -> (x*y=w248:dbl)
            n100 = Multiply(x=w241, y=w242) -> (x*y=w247:dbl)
            n101 = Bundle By Name(cluster=w227, "X Scale Width %"=w247, "Y Scale Height %"=w248) -> (w226:T6)
          }
          frame "[Scale] Align Scale Labels" {
            w276 = u32 2 ("y")
            n102 = property on="Property Node" class="WFGraph (strict)"(reference=w249) -> (reference out=w250:refnum<vi>, "Plot Bounds"=w262:T11, "XScale.NameLbl.Width"=w255:u32, "YScale.NameLbl.Height"=w259:u32)  [unwired: 1 in, 1 out]
            n103 = Unbundle By Name(w251) -> ("Amp Width"=w267:u32, "Amp Height"=w268:u32, "Z Height"=w274:u32)
            n104 = property on="Property Node" class="WFGraph (strict)"(reference=w252) -> (reference out=w253:refnum<vi>, "Plot Bounds"=w271:T11, "YScale.NameLbl.Height"=w275:u32)  [unwired: 1 in, 1 out]
            n105 = Unbundle By Name(w262) -> ("Top"=w263:i16, "Left"=w261:i16)
            n106 = Subtract(x=w267, y=w255) -> (x-y=w265:u32)
            n107 = Subtract(x=w268, y=w259) -> (x-y=w258:u32)
            n108 = To Long Integer(number=w265) -> (32bit integer=w266:i32)
            n109 = To Long Integer(number=w258) -> (32bit integer=w264:i32)
            n110 = Unbundle By Name(w271) -> ("Top"=w273:i16)
            n111 = Divide(x=w266, y=w276) -> (x/y=w254:dbl)
            n112 = Add(x=w261, y=w254) -> (x+y=w256:dbl)
            n113 = Subtract(x=w274, y=w275) -> (x-y=w270:u32)
            n114 = To Long Integer(number=w270) -> (32bit integer=w269:i32)
            n115 = Divide(x=w264, y=w276) -> (x/y=w257:dbl)
            n116 = Divide(x=w269, y=w276) -> (x/y=w272:dbl)
            n117 = Add(x=w263, y=w257) -> (x+y=w260:dbl)
            n118 = Add(x=w273, y=w272) -> (x+y=w277:dbl)
            n119 = property on="Property Node" class="WFGraph (strict)"(reference=w253, "YScale.NameLbl.Top"=w277) -> ()  [unwired: 1 in, 2 out]
            n120 = property on="Property Node" class="WFGraph (strict)"(reference=w250, "XScale.NameLbl.Left"=w256, "YScale.NameLbl.Top"=w260) -> ()  [unwired: 1 in, 2 out]
          }
          frame "[Plot] Initialize Plot" {
            n121 = Unbundle By Name(w286) -> ("X-Scale Visible"=w303:bool, "Y-Scale Visible"=w302:bool, "X-Axis Scaling Factor.Multiplier"=w300:dbl, "Y-Axis Scaling Factor.Multiplier"=w299:dbl, "X-Axis Name"=w291:string, "Y-Axis Name"=w292:string, "X-Axis Range Scaled.Minimum"=w293:dbl, "X-Axis Range Scaled.Maximum"=w294:dbl, "Y-Axis Range Scaled.Minimum"=w295:dbl, "Y-Axis Range Scaled.Maximum"=w296:dbl, "X-Scale Label Visible"=w307:bool, "Y-Scale Label Visible"=w306:bool, "X-Scale Format Str"=w308:string, "Y-Scale Format Str"=w309:string, "Z-Scale Visible"=w304:bool, "Z-Axis Range Scaled.Minimum"=w297:dbl, "Z-Axis Range Scaled.Maximum"=w298:dbl, "Z-Axis Name"=w301:string, "Z-Scale Label Visible"=w305:bool, "Z-Scale Format Str"=w310:string, "Z-Axis Scaling Factor.Multiplier"=w312:dbl)
            n122 = Less Than 0?(x=w300) -> (x < 0?=w289:bool)
            n123 = Less Than 0?(x=w312) -> (x < 0?=w311:bool)
            n124 = Less Than 0?(x=w299) -> (x < 0?=w290:bool)
            n125 = property on="Property Node" class="WFGraph (strict)"(reference=w288, "XScale.Visible"=w303, "YScale.Visible"=w302, "XScale.Flipped"=w289, "YScale.Flipped"=w290, "XScale.NameLbl.Text"=w291, "YScale.NameLbl.Text"=w292, "XScale.Minimum"=w293, "XScale.Maximum"=w294, "YScale.Minimum"=w295, "YScale.Maximum"=w296, "XScale.NameLbl.Visible"=w307, "YScale.NameLbl.Visible"=w306, "XScale.FormatString"=w308, "YScale.FormatString"=w309) -> ()  [unwired: 1 in, 2 out]
            n126 = property on="Property Node" class="WFGraph (strict)"(reference=w285, "YScale.Visible"=w304, "YScale.Minimum"=w297, "YScale.Maximum"=w298, "YScale.NameLbl.Text"=w301, "YScale.NameLbl.Visible"=w305, "YScale.FormatString"=w310, "YScale.Flipped"=w311) -> ()  [unwired: 1 in, 2 out]
          }
          frame "[Scale] X Scale" {
            n127 = Unbundle By Name(w314) -> ("X-Axis Range Scaled.Minimum"=w316:dbl, "X-Axis Range Scaled.Maximum"=w317:dbl)
            n128 = property on="Property Node" class="WFGraph (strict)"(reference=w315, "XScale.Minimum"=w316, "XScale.Maximum"=w317) -> ()  [unwired: 1 in, 2 out]
          }
          frame "[Scale] Y Scale" {
            n129 = Unbundle By Name(w322) -> ("Y-Axis Range Scaled.Minimum"=w325:dbl, "Y-Axis Range Scaled.Maximum"=w326:dbl)
            n130 = property on="Property Node" class="WFGraph (strict)"(reference=w324, "YScale.Minimum"=w325, "YScale.Maximum"=w326) -> ()  [unwired: 1 in, 2 out]
          }
          frame "[Scale] Z Scale" {
            n131 = Unbundle By Name(w331) -> ("Z-Axis Range Scaled.Minimum"=w334:dbl, "Z-Axis Range Scaled.Maximum"=w335:dbl)
            n132 = property on="Property Node" class="WFGraph (strict)"(reference=w333, "YScale.Minimum"=w334, "YScale.Maximum"=w335) -> ()  [unwired: 1 in, 2 out]
          }
          frame "[Scale] Multiplier/Offset" {
            n133 = Unbundle By Name(w342) -> ("X-Axis Scaling Factor.Multiplier"=w351:dbl, "Y-Axis Scaling Factor.Multiplier"=w350:dbl, "X-Axis Range Scaled.Minimum"=w345:dbl, "X-Axis Range Scaled.Maximum"=w352:dbl, "Y-Axis Range Scaled.Minimum"=w346:dbl, "Y-Axis Range Scaled.Maximum"=w347:dbl, "Z-Axis Range Scaled.Minimum"=w348:dbl, "Z-Axis Range Scaled.Maximum"=w349:dbl, "Z-Axis Scaling Factor.Multiplier"=w354:dbl)
            n134 = Less Than 0?(x=w351) -> (x < 0?=w343:bool)
            n135 = Less Than 0?(x=w354) -> (x < 0?=w353:bool)
            n136 = Less Than 0?(x=w350) -> (x < 0?=w344:bool)
            n137 = property on="Property Node" class="WFGraph (strict)"(reference=w341, "XScale.Flipped"=w343, "YScale.Flipped"=w344, "XScale.Minimum"=w345, "XScale.Maximum"=w352, "YScale.Minimum"=w346, "YScale.Maximum"=w347) -> ()  [unwired: 1 in, 2 out]
            n138 = property on="Property Node" class="WFGraph (strict)"(reference=w340, "YScale.Minimum"=w348, "YScale.Maximum"=w349, "YScale.Flipped"=w353) -> ()  [unwired: 1 in, 2 out]
          }
          frame "[Scale] Name" {
            n139 = Unbundle By Name(w362) -> ("X-Axis Name"=w363:string, "Y-Axis Name"=w364:string, "Z-Axis Name"=w365:string)
            n140 = property on="Property Node" class="WFGraph (strict)"(reference=w361, "XScale.NameLbl.Text"=w363, "YScale.NameLbl.Text"=w364) -> ()  [unwired: 1 in, 2 out]
            n141 = property on="Property Node" class="WFGraph (strict)"(reference=w360, "YScale.NameLbl.Text"=w365) -> ()  [unwired: 1 in, 2 out]
          }
          frame "[Scale] Visible" {
            n142 = Unbundle By Name(w373) -> ("X-Scale Visible"=w374:bool, "Y-Scale Visible"=w375:bool, "Z-Scale Visible"=w376:bool)
            n143 = property on="Property Node" class="WFGraph (strict)"(reference=w372, "XScale.Visible"=w374, "YScale.Visible"=w375) -> ()  [unwired: 1 in, 2 out]
            n144 = property on="Property Node" class="WFGraph (strict)"(reference=w371, "YScale.Visible"=w376) -> ()  [unwired: 1 in, 2 out]
          }
          frame "[Scale] Label Visible" {
            n145 = Unbundle By Name(w382) -> ("X-Scale Label Visible"=w386:bool, "Y-Scale Label Visible"=w387:bool, "Z-Scale Label Visible"=w388:bool)
            n146 = property on="Property Node" class="WFGraph (strict)"(reference=w384, "XScale.NameLbl.Visible"=w386, "YScale.NameLbl.Visible"=w387) -> ()  [unwired: 1 in, 2 out]
            n147 = property on="Property Node" class="WFGraph (strict)"(reference=w383, "YScale.NameLbl.Visible"=w388) -> ()  [unwired: 1 in, 2 out]
          }
          frame "[Scale] Format" {
            n148 = Unbundle By Name(w395) -> ("X-Scale Format Str"=w396:string, "Y-Scale Format Str"=w397:string, "Z-Scale Format Str"=w398:string)
            n149 = property on="Property Node" class="WFGraph (strict)"(reference=w394, "XScale.FormatString"=w396, "YScale.FormatString"=w397) -> ()  [unwired: 1 in, 2 out]
            n150 = property on="Property Node" class="WFGraph (strict)"(reference=w393, "YScale.FormatString"=w398) -> ()  [unwired: 1 in, 2 out]
          }
        }
      }
      n151 = property class="Pnl"(reference=w27, error in=w28, "DeferPanUpdts"=FALSE ("Defer Panel Updates")) -> ()  [unwired: 2 out]
    }
    frame True {
    }
  }
  "Display State Out" <- w8
  "Data Out" <- w9
  "Dec/Cropped out" <- w6
